vi "ma_In Range Utility.vi"(1 "low":dbl format="%0.2f", 2 "x":dbl format="%0.2f", 3 "high":dbl format="%0.2f") -> (0 "lo <= x <=  hi?":bool)   [LabVIEW 2020, in "NI_MAPro.lvlib"]
uses:
  NI_MAPro.lvlib
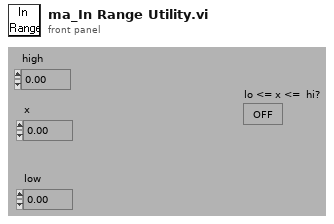
[diagram p1: front panel]
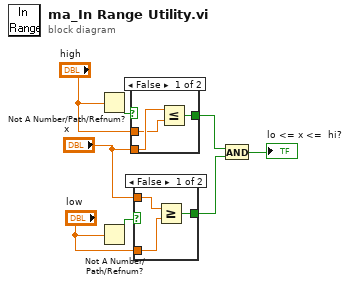
[diagram p0: block diagram]
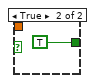
[diagram p2: hidden frame]
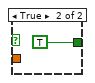
[diagram p3: hidden frame]
diagram:
  n1 = Not A Number/Path/Refnum?(number/path/refnum="high") -> (NaN/Path/Refnum?=w4:bool)
  n2 = Not A Number/Path/Refnum?(number/path/refnum="low") -> (NaN/Path/Refnum?=w3:bool)
  n3 = case shown="False" w4 {
    tunnel: "x" -> [w10 _]
    tunnel: [w11 TRUE] -> w7
    tunnel: "high" -> [w9 _]
    frame False {
      n4 = Less Or Equal?(x=w10, y=w9) -> (x <= y?=w11:bool)
    }
    frame True {
    }
  }
  n5 = case shown="False" w3 {
    tunnel: "x" -> [w15 _]
    tunnel: [w14 TRUE] -> w6
    tunnel: "low" -> [w13 _]
    frame False {
      n6 = Greater Or Equal?(x=w15, y=w13) -> (x >= y?=w14:bool)
    }
    frame True {
    }
  }
  n7 = And(x=w7, y=w6) -> (x .and. y?=→"lo <= x <=  hi?":bool)
